vi "Remove_SbPnl.vi"(0 "reference in":refnum<class "GUI.lvclass">, 5 "error in (no error)":errorcluster) -> (14 "reference out":refnum<class "GUI.lvclass">, 19 "error out":errorcluster)   [LabVIEW 2019, in "GUI.lvclass"]
uses:
  GUI.lvclass
  GUI.lvclass/GUI.ctl
  WindowsState.ctl
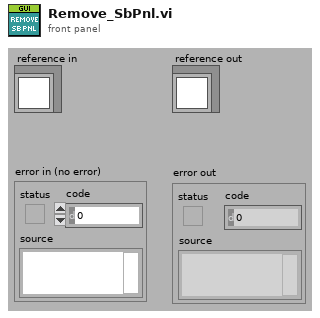
[diagram p1: front panel]
types:
  T1 = typedef "GUI.lvclass/WindowsState.ctl" = enum16{"NotReady", "Ready", "Inserted", "Opened"}
  T2 = typedef "GUI.lvclass/Shered Data.ctl" = cluster{"WindowsState":T1, "UI VI":refnum<vi>, "SubPnl":refnum<vi>}
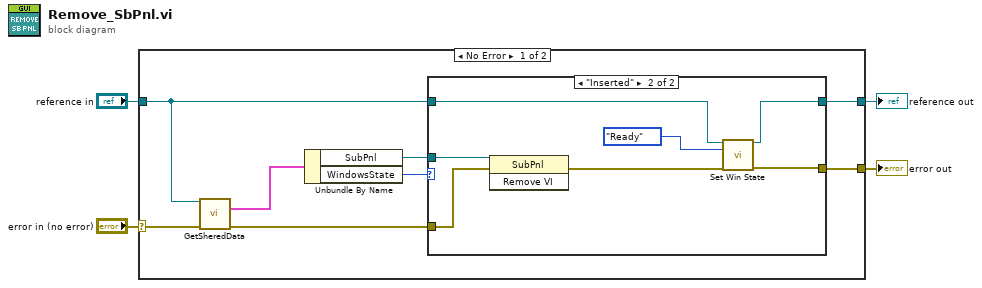
[diagram p0: block diagram]
diagram:
  n1 = case shown="No Error" "error in (no error)" {
    selector: "error in (no error)" -> [w7 w23]
    tunnel: [w12 w23] -> w3
    tunnel: [w11 w22] -> w1
    tunnel: "reference in" -> [w10 w22]
    frame No Error {
      n2 = call "GetSheredData.vi"("reference in"=w10, "error in (no error)"=w7) -> ("data"=w9:T2, "error out"=w6:errorcluster)  [unwired: 11 in, 1 out]
      n3 = Unbundle By Name(w9) -> ("SubPnl"=w5:refnum<vi>, "WindowsState"=w8:T1)
      n4 = case shown="\"Inserted\"" w8 {
        tunnel: w5 -> [_ w21]
        tunnel: w6 -> [w14 w20]
        tunnel: [w14 w16] -> w12
        tunnel: w10 -> [w13 w19]
        tunnel: [w13 w15] -> w11
        frame Default {
        }
        frame "Inserted" {
          n5 = invoke class="SubPnl" method="Remove VI"(reference=w21, error in=w20) -> (error out=w17:errorcluster)  [unwired: 1 in, 2 out]
          n6 = call "Set Win State.vi"("reference in"=w19, "WindowsState"=WindowsState."Ready", "error in (no error)"=w17) -> ("reference out"=w15:refnum<class "GUI.lvclass">, "error out"=w16:errorcluster)  [unwired: 11 in]
        }
      }
    }
    frame Error {
    }
  }
  "error out" <- w3
  "reference out" <- w1
